vi "Konfig Leak Check.vi"() -> ()   [LabVIEW 2020, in "EPA 1065.lvlib" / "Dichtheitstest 1065-345.lvlib"]
uses:
  Dichtheitstest 1065-345.lvlib
  VFS Button.ctl
  HL Button.ctl
  Versa Button.ctl
  Visualisierungs Elemente/Zahlen-Ausgabefeld.ctl
  Leak Protokoll Einstellungen.ctl
  Seiten/System Einstellungen V2/Analysatoren.ctl
  Aktion Leak Daten.ctl
  Aktion Leak check durchfuehren.ctl
  Aktion Protokolldaten_Leak check.ctl
  Sprachverwaltung/FGV Aktion Tabelle zerlegen.ctl
  Aktion FGV Automatic start.ctl
  Allgemeine VIs/Aktion Wertaenderung Gasliste.ctl
  Allgemeine VIs/Aktion Test Status.ctl
  PNS/Aktionen FGV Grenzwerte.ctl
  Funktionstasten/Zustaende.ctl
  Allgemein/allgemeine Sub-VIs.lvlib
  PNS/PNS.lvlib
  Funktionstasten/Funktionstasten.lvlib
  Sprachverwaltung/Sprachverwaltung.lvlib
  EPA 1065.lvlib
  Linearisierung V2/Protokoll/Protokoll.lvlib
  Seiten/System Einstellungen V2/System Einstellungen V2.lvlib
panel:
  out "Einheit Ergebnis":string caption="Einheit"
  out "Einheit Grenze":string caption="Einheit"
  in  "Einheit":enum16{"mol/s", "mbar"}(ring) caption="Unit:"
  in  "LeakValve":u16(ring) caption="Leak Valve:" items=["inactive", "active"]
  in  "Systemeinstellung":bool caption="Gasliste geändert"
  in  "Save to file":bool caption="Speichern"
  in  "Werte Speichern":bool
  in  "Heizleitung zum VFS":bool caption="Heizleitung\nzum\nVFS"
  in  "HL zu VFS button":T1
  in  "Länge HL zu SP":sgl caption="mm" format="%#.5f"
  in  "Innendurchmesser \nHL zu SP":sgl caption="mm" format="%#.5f"
  in  "Gesamtvolumen VFS":sgl caption="mm³" format="%#.5f"
  in  "Länge HL zu VFS":sgl caption="mm" format="%#.5f"
  in  "Innendurchmesser \nHL zu VFS":sgl caption="mm" format="%#.5f"
  in  "Gesamtvolumen FAS":sgl caption="mm³" format="%#.5f"
  in  "Heizleitung zur Entnahmestelle":bool caption="Heizleitung\nzur\nEntnahmestelle"
  in  "VFS":bool
  in  "HL zu SP button":T1
  in  "VFS button":T2
  out "Anzeige":string
  out "Ergebnis":sgl format="%#.8f"
  out "Grenzwert":sgl format="%#.8f"
  in  "Abbrechen":bool
  in  "Start":bool
  out "Druckanstieg:":T3 caption="mbar"
  out "Druck FT-IR:":T3 caption="atm" format="%.3f"
  out "Status:":string
  in  "Textname:":string
  in  "Pfad:":path=path "D:/IAG_Data"
  in  "PDF speichern":bool caption="Speichern"
  in  "Leak Protokoll":T4={"Bearbeiter:"="", "Pfad:"=path "D:/IAG_Data/Log", "Textname:"="", "Analysator"=""}
  in  "FAS button":T6
  # "Volumen-Einstellungen"
  # "Status"
  # "Druck FT-IR:"
  # "Druckanstieg:"
  # "Innendurchmesser \nHL zu VFS"
  # "Innendurchmesser \nHL zu SP"
  # "Gesamtvolumen Versa"
  # "Gesamtvolumen VFS"
  # "Länge HL zu VFS"
  # "Länge HL zu SP"
  # "Dichtheitstest EPA CRF40 §1065.345"
  # "Protokolleinstellungen"
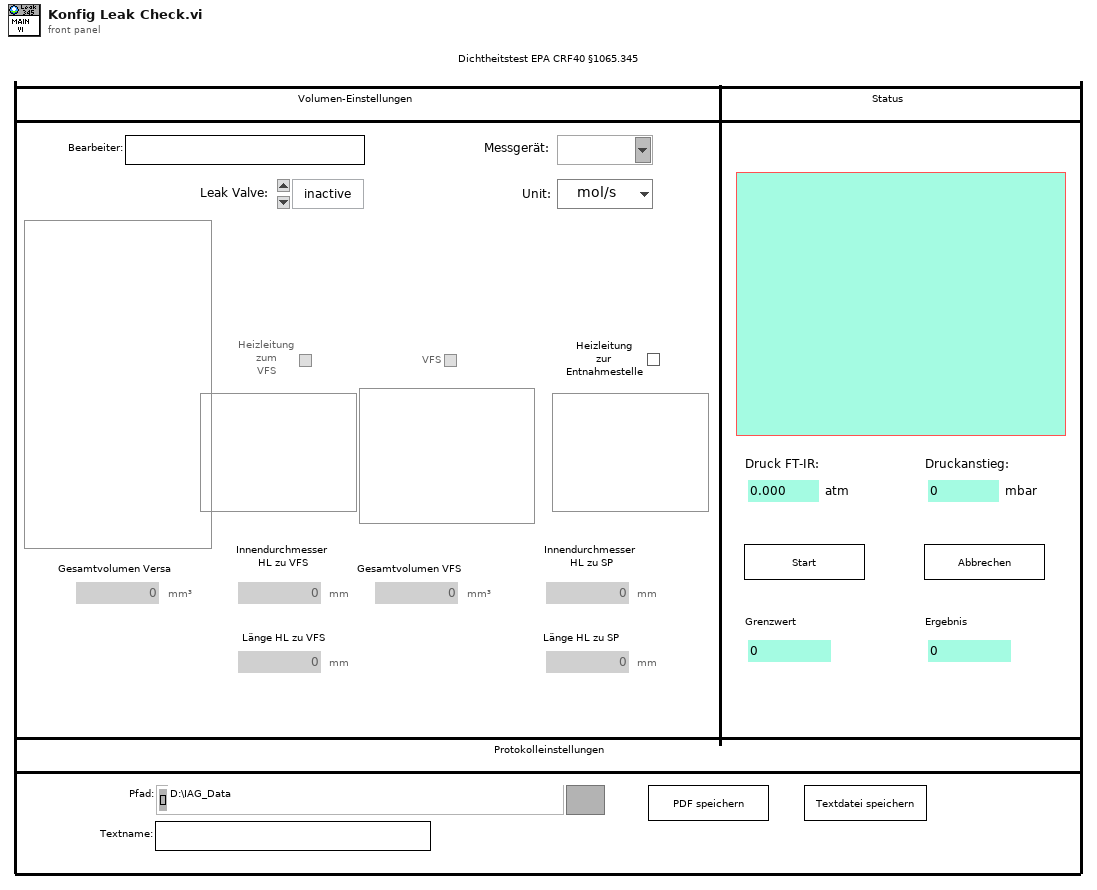
[diagram p1: front panel]
types:
  T1 = typedef "EPA 1065.lvlib/Dichtheitstest 1065-345.lvlib/HL Button.ctl" = bool
  T2 = typedef "EPA 1065.lvlib/Dichtheitstest 1065-345.lvlib/VFS Button.ctl" = bool
  T3 = typedef "Zahlen-Ausgabefeld.ctl" = sgl
  T4 = typedef "EPA 1065.lvlib/Dichtheitstest 1065-345.lvlib/Leak Protokoll Einstellungen.ctl" = cluster{"Bearbeiter:":string, "Pfad:":path, "Textname:":string, "Analysator":T5}
  T5 = typedef "System Einstellungen V2.lvlib/Analysatoren.ctl" = string
  T6 = typedef "EPA 1065.lvlib/Dichtheitstest 1065-345.lvlib/Versa Button.ctl" = bool
  T7 = typedef "Sprachverwaltung.lvlib/FGV Aktion Tabelle zerlegen.ctl" = enum16{"laden", "vereinzeln", "speichern"}
  T8 = typedef "EPA 1065.lvlib/Dichtheitstest 1065-345.lvlib/Aktion Protokolldaten_Leak check.ctl" = enum16{"lesen", "Zeitstempel", "Bearbeiter", "Daten", "Auswertung", "löschen"}
  T9 = typedef "EPA 1065.lvlib/Dichtheitstest 1065-345.lvlib/Aktion Leak Daten.ctl" = enum16{"lesen", "laden", "speichern", "Volumen", "berechnen", "Leak check aktiv", "Leak Zustand", "Pfad", "Pfad speichern"}
  T10 = typedef "EPA 1065.lvlib/Dichtheitstest 1065-345.lvlib/Aktion Leak check durchfuehren.ctl" = enum16{"initialisieren", "Unterdruck erzeugen", "Ventile schließen", "Warten", "Auswertung", "fertig", "PDF erstellen", "abbrechen"}
  T11 = enum8{"Enabled", "Disabled", "Disabled and Grayed Out"}
  T12 = typedef "EPA 1065.lvlib/Dichtheitstest 1065-345.lvlib/Aktion FGV Automatic start.ctl" = enum16{"lesen", "Test starten aktiv", "Test starten inaktiv", "Seite merken", "Seite zurücksetzen", "AK Start inaktiv"}
  T13 = typedef "EPA 1065.lvlib/Dichtheitstest 1065-345.lvlib/Gesamtvolumen.ctl" = cluster{"FAS":sgl, "d von HL zu VFS":sgl, "l von HL zu VFS":sgl, "VFS":sgl, "d von HL zu SP":sgl, "l von HL zu SP":sgl, "Heizleitung zum VFS":bool, "VFS a":bool, "Heizleitung zur Entnahmestelle":bool, "Gesamtes Volumen":sgl, "LeakValve":u16, "Einheit":enum16{"mol/s", "mbar"}}
  T14 = typedef "EPA 1065.lvlib/Aktion Wertaenderung Gasliste.ctl" = enum16{"Init", "lesen", "Gasliste geändert", "ARN inaktiv", "LEAK inaktiv", "Interference 366 inaktiv", "T90 inaktiv", "Interference 375 inaktiv", "Chiller inaktiv", "FID O2 inaktiv", "FID Opti inaktiv", "Drift inaktiv", "Pre Test inaktiv", "LinV2 inaktiv", "HovaCAL Interference inaktiv"}
  T15 = typedef "EPA 1065.lvlib/Aktion Test Status.ctl" = enum16{"init", "lesen", "prüfen", "Interference 366", "Interference 375", "Chiller läuft", "Drift läuft", "Pre Test läuft", "FID Optimization läuft", "FID Interference läuft", "HovaCAL Interference", "LinV2"}
  T16 = enum16{"open", "replace", "create", "open or create", "replace or create", "replace or create with confirmation"}
  T17 = typedef "Funktionstasten.lvlib/Zustaende.ctl" = enum16{"Standby", "Pause", "Eco", "Messen", "Kalibrieren", "Spülen Filter", "Spülen Leitung", "Umgebungsluft", "0-Gas", "Cal-Gas", "CG zu PNS", "-------------", "Init 1", "Init 2", "Init 3", "Init 4", "Messen vorbereiten", "Messen durchführen", "Exit"}
  T18 = typedef "PNS.lvlib/Aktionen FGV Grenzwerte.ctl" = enum16{"lesen", "Grenzw. schreiben", "Anweisungscode", "IP-Adresse", "laden", "speichern", "Anweisungscode vorgeben"}
  T19 = typedef "EPA 1065.lvlib/Dichtheitstest 1065-345.lvlib/Leak Daten.ctl" = cluster{"Gesamtes Volumen":sgl, "p 1":sgl, "p 2":sgl, "T 1":sgl, "T 2":sgl, "t 1":timestamp, "t 2":timestamp, "Ergebnis mol/s":sgl, "Grenze mol/s":sgl, "Leak in %":sgl, "Ergebnis mbar":sgl, "Grenze mbar":sgl}
  T20 = typedef "EPA 1065.lvlib/Aktive Tests Cluster.ctl" = cluster{"ANR läuft":bool, "T90 läuft":bool, "Leak läuft":bool, "Interference 366 läuft":bool, "Interference 375 läuft":bool, "Chiller läuft":bool, "FID Interference läuft":bool, "FID optimization läuft":bool, "Drift läuft":bool, "Pre-test läuft":bool, "HovaCAL Interference läuft":bool, "LinV2 läuft":bool}
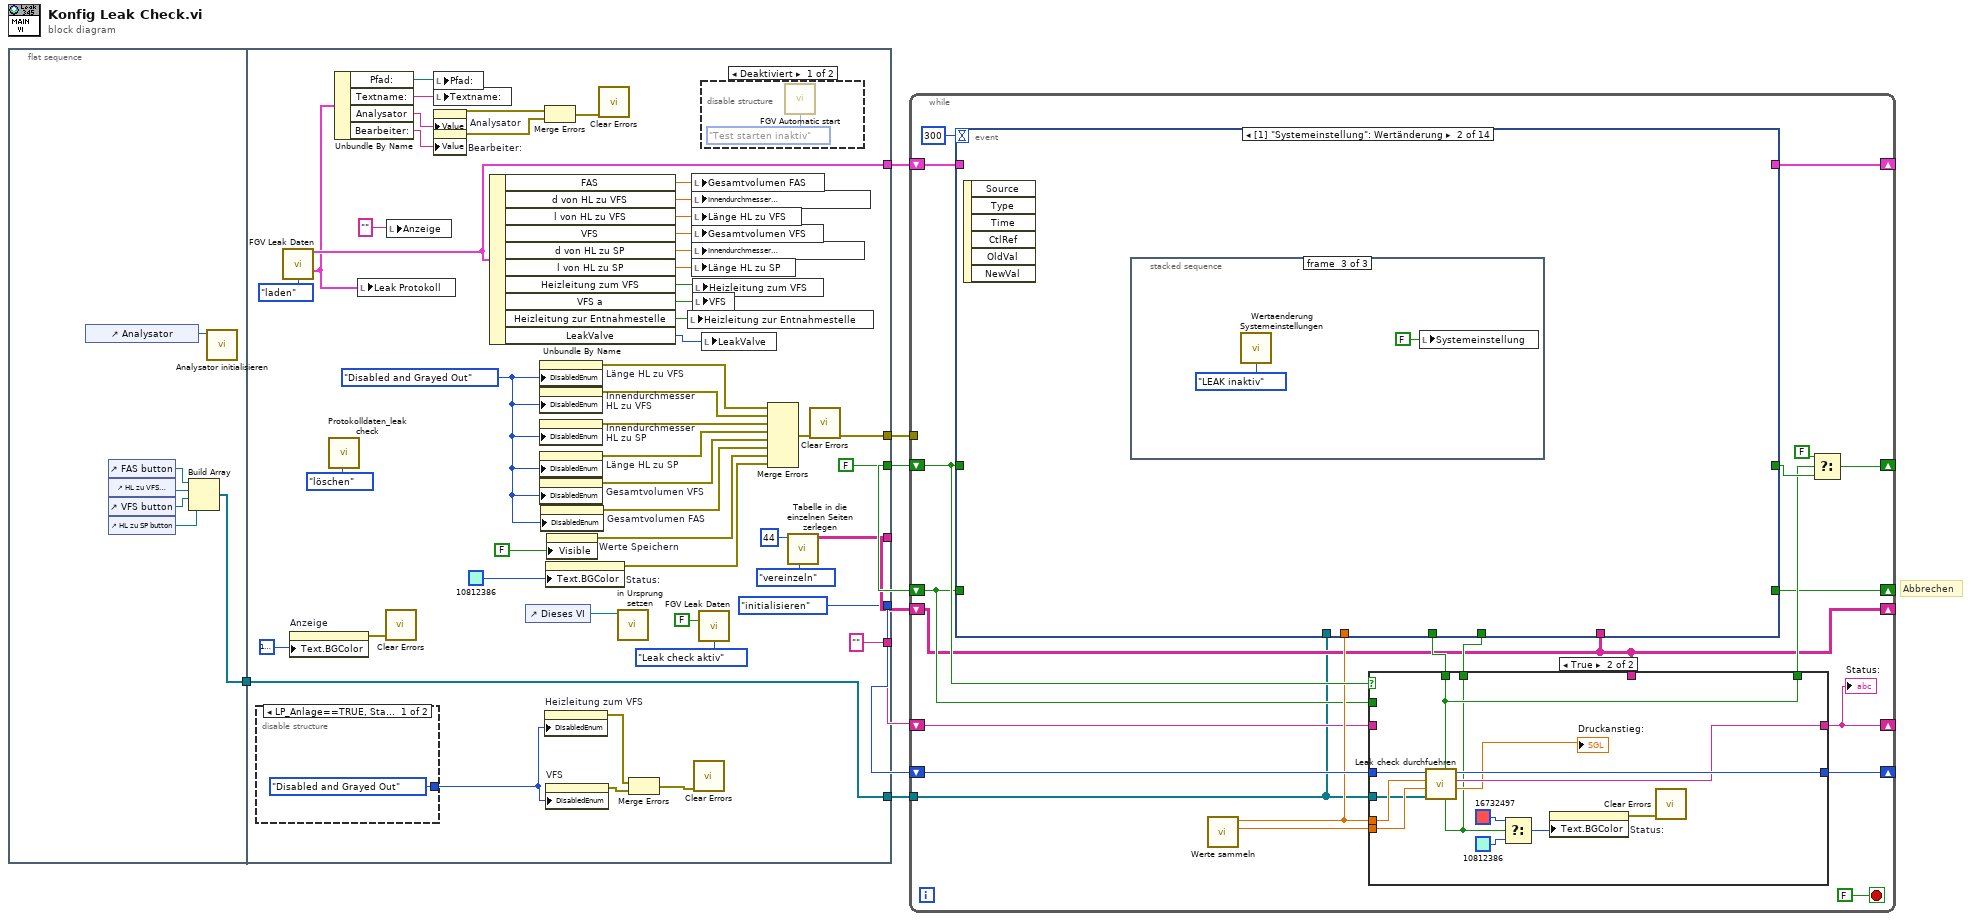
[diagram p0: block diagram]
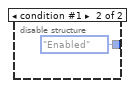
[diagram p2: hidden frame]
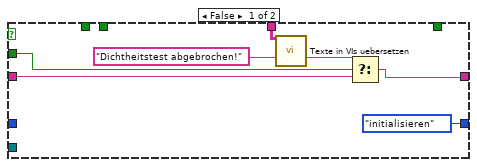
[diagram p4: hidden frame]
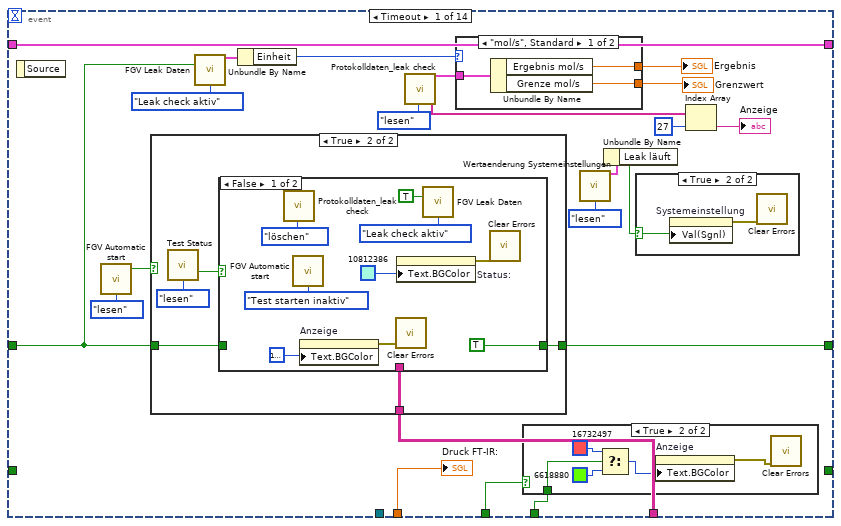
[diagram p5: hidden frame]
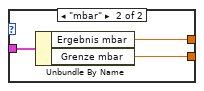
[diagram p6: hidden frame]
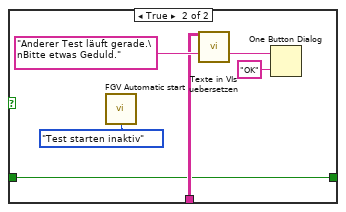
[diagram p9: hidden frame]
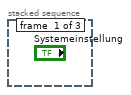
[diagram p11: hidden frame]
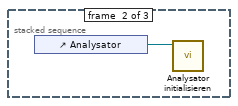
[diagram p12: hidden frame]
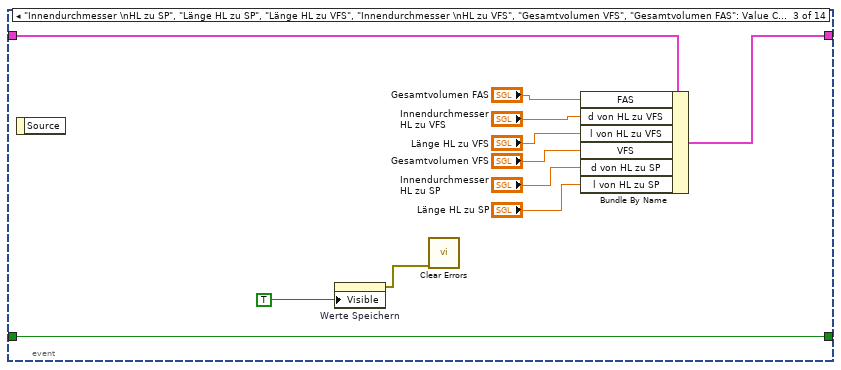
[diagram p13: hidden frame]
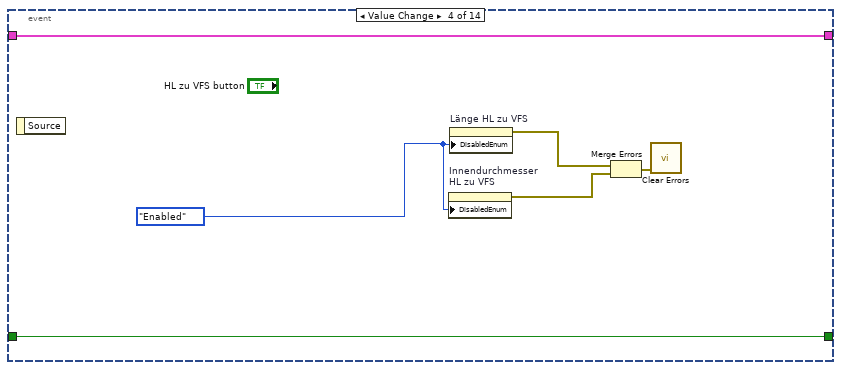
[diagram p14: hidden frame]
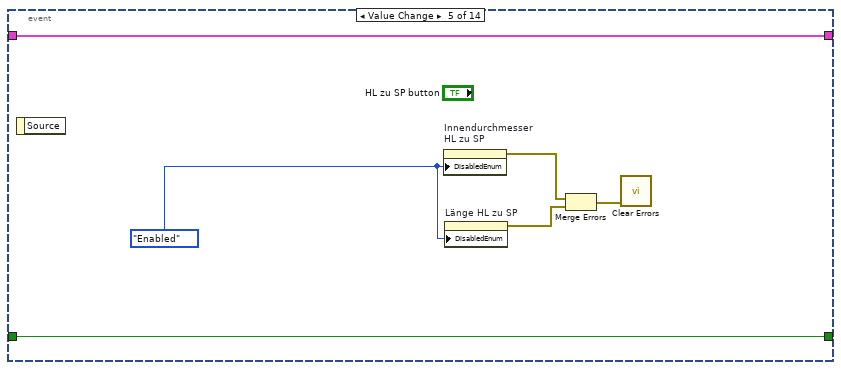
[diagram p15: hidden frame]
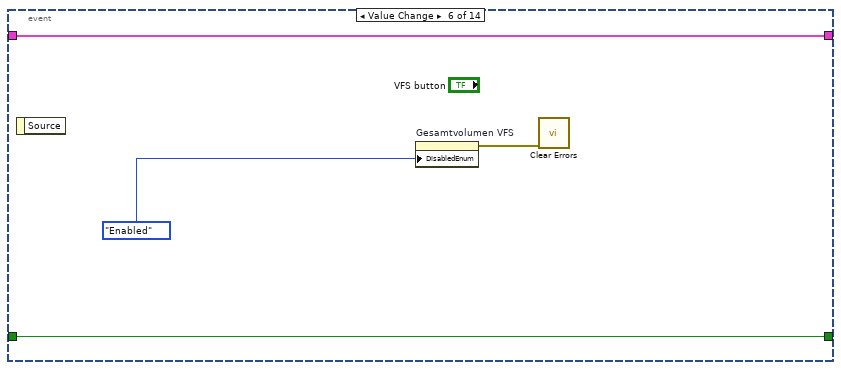
[diagram p16: hidden frame]
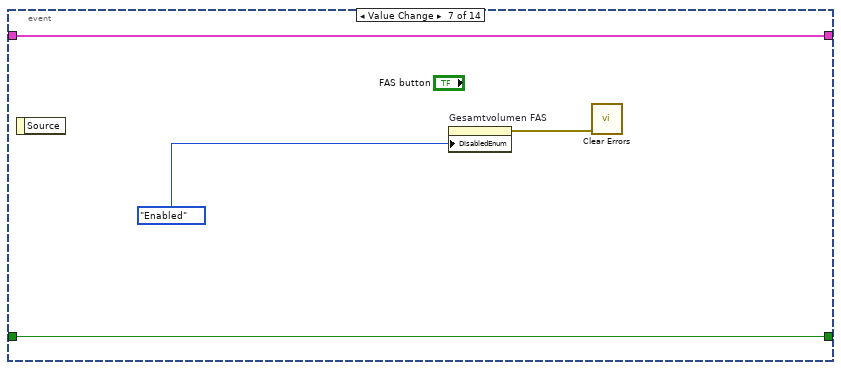
[diagram p17: hidden frame]
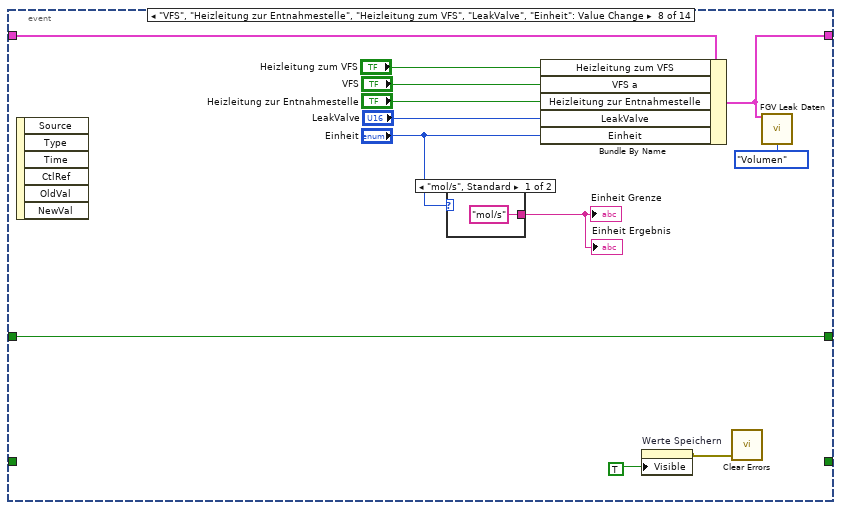
[diagram p18: hidden frame]
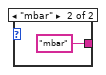
[diagram p19: hidden frame]
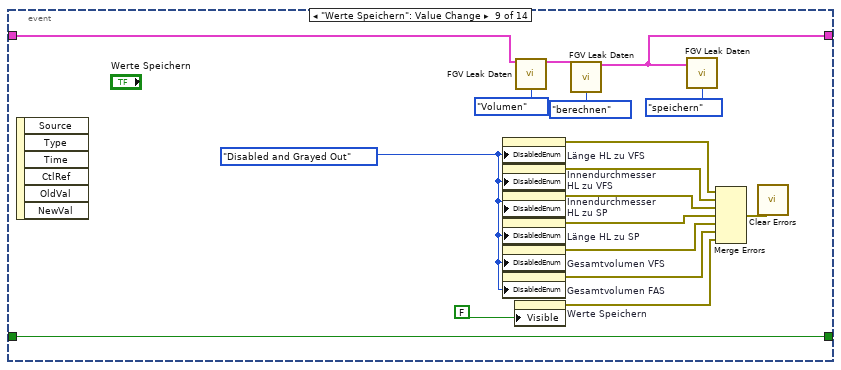
[diagram p20: hidden frame]
diagram:
  # "Abbrechen"
  n1 = flat-sequence {
    tunnel: [w9] -> w2
    tunnel: [w59] -> w8
    tunnel: [w46] -> w7
    tunnel: [FALSE] -> w4
    tunnel: [Aktion_Leak_check_durchfuehren."initialisieren" ("Aktion")] -> w6
    tunnel: ["" ("Status")] -> w5
    tunnel: [w32] -> w3
    tunnel: w2 -> [w15]
    tunnel: [w15] -> w1
    frame #0 {
      n2 = control-ref of="Analysator"() -> (w14:refnum<vi>)
      n3 = control-ref of="FAS button"() -> (w13:refnum<vi>)
      n4 = control-ref of="HL zu VFS button"() -> (w12:refnum<vi>)
      n5 = control-ref of="VFS button"() -> (w11:refnum<vi>)
      n6 = control-ref of="HL zu SP button"() -> (w10:refnum<vi>)
      n7 = Build Array(w13, w12, w11, w10) -> (w9:refnum<vi>[])
      n8 = call "Analysator initialisieren.vi"("Referenz Analysator"=w14) -> ()  [unwired: 9 in, 2 out]
    }
    frame #1 {
      w38 = T11."Disabled and Grayed Out" ("Deaktiviert")
      n9 = disable-structure shown="LP_Anlage==TRUE, Standard" {
        disable-tunnel: [T11."Disabled and Grayed Out" ("Deaktiviert") T11."Enabled" ("Deaktiviert")] -> w20
        frame condition #0 (active) {
        }
        frame condition #1 {
        }
      }
      n10 = call "FGV Leak Daten.vi"("Aktion"=Aktion_Leak_Daten."laden") -> ("Gesamtvolumen"=w46:T13, "Leak Protokoll"=w28:T4)  [unwired: 10 in, 3 out]
      n11 = property on="Anzeige" class="Str"("Text.BGColor"=u32 16777216) -> (error out=w34:errorcluster)  [unwired: 2 in, 1 out]
      n12 = call "Protokolldaten_leak check.vi"("Aktion"=Aktion_Protokolldaten_Leak_check."löschen") -> ()  [unwired: 23 in, 4 out]
      n13 = Unbundle By Name(w28) -> ("Pfad:"=w27:path, "Textname:"=w26:string, "Analysator"=w25:T5, "Bearbeiter:"=w24:string)
      n14 = local write "Leak Protokoll"(w28) -> ()
      n15 = call <vilib>:"Clear Errors.vi"("error in (no error)"=w34) -> ()  [unwired: 5 in, 2 out]
      n16 = local write "Anzeige"("" ("Anzeige")) -> ()
      n17 = local write "Pfad:"(w27) -> ()
      n18 = local write "Textname:"(w26) -> ()
      n19 = property on="Analysator" class="KombiFeld (strikt)"("Value"=w25) -> (error out=w22:errorcluster)  [unwired: 2 in, 1 out]
      n20 = property on="Bearbeiter:" class="Str"("Value"=w24) -> (error out=w21:errorcluster)  [unwired: 2 in, 1 out]
      n21 = Unbundle By Name(w46) -> ("FAS"=w55:sgl, "d von HL zu VFS"=w53:sgl, "l von HL zu VFS"=w52:sgl, "VFS"=w51:sgl, "d von HL zu SP"=w50:sgl, "l von HL zu SP"=w54:sgl, "Heizleitung zum VFS"=w48:bool, "VFS a"=w47:bool, "Heizleitung zur Entnahmestelle"=w49:bool, "LeakValve"=w16:u16)
      n22 = control-ref of="Dieses VI"() -> (w57:refnum<vi>)
      n23 = property on="Länge HL zu VFS" class="DigWert (strikt)"("DisabledEnum"=w38) -> (error out=w64:errorcluster)  [unwired: 2 in, 1 out]
      n24 = property on="Innendurchmesser \nHL zu VFS" class="DigWert (strikt)"("DisabledEnum"=w38) -> (error out=w63:errorcluster)  [unwired: 2 in, 1 out]
      n25 = property on="Innendurchmesser \nHL zu SP" class="DigWert (strikt)"("DisabledEnum"=w38) -> (error out=w62:errorcluster)  [unwired: 2 in, 1 out]
      n26 = property on="Länge HL zu SP" class="DigWert (strikt)"("DisabledEnum"=w38) -> (error out=w61:errorcluster)  [unwired: 2 in, 1 out]
      n27 = property on="Gesamtvolumen VFS" class="DigWert (strikt)"("DisabledEnum"=w38) -> (error out=w60:errorcluster)  [unwired: 2 in, 1 out]
      n28 = property on="Gesamtvolumen FAS" class="DigWert (strikt)"("DisabledEnum"=w38) -> (error out=w58:errorcluster)  [unwired: 2 in, 1 out]
      n29 = Merge Errors(w22, w21) -> (w23:errorcluster)
      n30 = property on="Heizleitung zum VFS" class="Bool. (strikt)"("DisabledEnum"=w20) -> (error out=w18:errorcluster)  [unwired: 2 in, 1 out]
      n31 = property on="Status:" class="Str"("Text.BGColor"=u32 10812386 ("Hintergrund")) -> (error out=w39:errorcluster)  [unwired: 2 in, 1 out]
      n32 = property on="VFS" class="Bool. (strikt)"("DisabledEnum"=w20) -> (error out=w19:errorcluster)  [unwired: 2 in, 1 out]
      n33 = property on="Werte Speichern" class="Bool."("Visible"=FALSE ("Sichtbar")) -> (error out=w30:errorcluster)  [unwired: 2 in, 1 out]
      n34 = call <vilib>:"Clear Errors.vi"("error in (no error)"=w23) -> ()  [unwired: 5 in, 2 out]
      n35 = call "in Ursprung setzen.vi"("VI Referenz"=w57) -> ()  [unwired: 10 in, 1 out]
      n36 = Merge Errors(w18, w19) -> (w17:errorcluster)
      n37 = local write "Heizleitung zur Entnahmestelle"(w49) -> ()
      n38 = local write "Gesamtvolumen FAS"(w55) -> ()
      n39 = local write "Innendurchmesser \nHL zu VFS"(w53) -> ()
      n40 = local write "Länge HL zu VFS"(w52) -> ()
      n41 = local write "Gesamtvolumen VFS"(w51) -> ()
      n42 = local write "Innendurchmesser \nHL zu SP"(w50) -> ()
      n43 = local write "Länge HL zu SP"(w54) -> ()
      n44 = local write "Heizleitung zum VFS"(w48) -> ()
      n45 = local write "VFS"(w47) -> ()
      n46 = call <vilib>:"Clear Errors.vi"("error in (no error)"=w17) -> ()  [unwired: 5 in, 2 out]
      n47 = call "FGV Leak Daten.vi"("Dichtheitstest aktiv"=FALSE, "Aktion"=Aktion_Leak_Daten."Leak check aktiv") -> ()  [unwired: 9 in, 5 out]
      n48 = disable-structure shown="Deaktiviert" {
        frame Disabled {
          n49 = call "FGV Automatic start.vi"("Aktion"=Aktion_FGV_Automatic_start."Test starten inaktiv") -> ()  [unwired: 12 in, 3 out]
        }
        frame Enabled {
        }
      }
      n50 = local write "LeakValve"(w16) -> ()
      n51 = Merge Errors(w64, w63, w62, w61, w60, w58, w30, w39) -> (w65:errorcluster)
      n52 = call "Tabelle in die einzelnen Seiten zerlegen.vi"("Aktion"=FGV_Aktion_Tabelle_zerlegen."vereinzeln", "Index (Seite)"=44) -> ("Sprachliste"=w32:string[][])  [unwired: 7 in, 2 out]
      n53 = call <vilib>:"Clear Errors.vi"("error in (no error)"=w65) -> ("error out"=w59:errorcluster)  [unwired: 5 in, 1 out]
    }
  }
  n54 = while {
    tunnel: w8 -> [_]
    shift-right: [w86] -> _
    shift-left: w7 -> [w87]
    shift-right: [w77] -> _
    shift-left: w4 -> [w85]
    shift-right: [w82] -> _
    shift-left: w6 -> [w83]
    shift-right: [w80] -> _
    shift-left: w5 -> [w79]
    shift-right: [w74] -> _
    shift-left: w4 -> [w73]
    shift-right: [w70] -> _
    shift-left: w3 -> [w70]
    tunnel: w1 -> [w69]
    stop <- FALSE stop-if-true
    n55 = call "Werte sammeln.vi"() -> ("Temperatur"=w84:sgl, "Druck FTIR"=w81:sgl)  [unwired: 10 in]
    n56 = case shown="True" w85 {
      tunnel: w81 -> [_ w109]
      tunnel: w84 -> [_ w108]
      tunnel: w83 -> [_ w107]
      tunnel: [Aktion_Leak_check_durchfuehren."initialisieren" ("Aktion") w106] -> w82
      tunnel: [w94 w105] -> w80
      tunnel: w79 -> [w93 _]
      tunnel: w73 -> [w95 _]
      tunnel: [_ w100] -> w75
      tunnel: [_ w100] -> w72
      tunnel: [_ w98] -> w71
      tunnel: w70 -> [w90 _]
      tunnel: w69 -> [_ w97]
      frame False {
        n57 = call "Texte in VIs uebersetzen.vi"("Sprachliste"=w90, "String zum Übersetzen"="Dichtheitstest abgebrochen!" ("t")) -> ("String zum Übersetzen"=w91:string)  [unwired: 9 in, 4 out]
        n58 = Select(t=w91, s=w95, f=w93) -> (s? t:f=w94:string)
      }
      frame True {
        n59 = call "Leak check durchfuehren.vi"("TablePictures Refnum In"=w97, "Temperatur"=w108, "Druck FT-IR"=w109, "Aktion"=w107) -> ("Druckanstieg"=→"Druckanstieg:":sgl, "Status"=w105:string, "Aktion"=w106:T10, "Fehler"=w98:bool, "Fertig"=w100:bool)  [unwired: 2 in, 1 out]
        n60 = Select(t=u32 16732497 ("Hintergrund"), s=w98, f=u32 10812386 ("Hintergrund")) -> (s? t:f=w102:u32)
        n61 = property on="Status:" class="Str"("Text.BGColor"=w102) -> (error out=w101:errorcluster)  [unwired: 2 in, 1 out]
        n62 = call <vilib>:"Clear Errors.vi"("error in (no error)"=w101) -> ()  [unwired: 5 in, 2 out]
      }
    }
    "Status:" <- w80
    n63 = event shown="[1] \"Systemeinstellung\": Wertänderung" {
      selector: _ -> [_ _ _ _ _ _ _ _ _ _ _ _ _ _]
      dyn-events: _ -> [_ _ _ _ _ _ _ _ _ _ _ _ _ _]
      timeout: 300 -> [_ _ _ _ _ _ _ _ _ _ _ _ _ _]
      tunnel: w87 -> [w129 _ w179 w182 w188 w194 w198 w211 w228 w246 w267 w293 w300 w322]
      tunnel: [w129 _ w178 w182 w188 w194 w198 w205 w218 w246 w267 w293 w300 w322] -> w86
      tunnel: w85 -> [w118 _ w171 w181 w187 w193 w197 w207 w217 w247 w266 w295 _ w320]
      tunnel: [w120 _ w171 w181 w187 w193 w197 w207 w217 w247 w266 w295 w299 w321] -> w78
      tunnel: w81 -> [w131 _ _ _ _ _ _ _ _ _ _ _ _ _]
      tunnel: [_ _ _ _ _ _ _ _ _ w248 w265 w294 _ w319] -> w74
      tunnel: w73 -> [_ _ _ _ _ _ _ _ _ w248 w265 w294 _ _]
      tunnel: w72 -> [w124 _ _ _ _ _ _ _ _ _ _ _ _ _]
      tunnel: w71 -> [w123 _ _ _ _ _ _ _ _ _ _ _ _ _]
      tunnel: w70 -> [w119 _ _ _ _ _ _ _ _ _ _ _ w296 _]
      tunnel: w69 -> [_ _ _ _ _ _ _ _ _ w231 _ _ _ _]
      event Timeout {
        n64 = event-data() -> ()  [unwired: 1 in, 1 out]
        n65 = call "FGV Automatic start.vi"("Aktion"=Aktion_FGV_Automatic_start."lesen") -> ("Starten"=w122:bool)  [unwired: 12 in, 2 out]
        n66 = case shown="True" w122 {
          tunnel: [w140 w143] -> w120
          tunnel: w119 -> [_ w142]
          tunnel: w118 -> [w140 w141]
          frame False {
          }
          frame True {
            n67 = call "Test Status.vi"("Aktion"=Aktion_Test_Status."lesen") -> ("Tests sperren"=w145:bool)  [unwired: 11 in, 3 out]
            n68 = case shown="False" w145 {
              tunnel: [TRUE w156] -> w143
              tunnel: w142 -> [_ w157]
              tunnel: w141 -> [_ w156]
              frame False {
                n69 = call "Protokolldaten_leak check.vi"("Aktion"=Aktion_Protokolldaten_Leak_check."löschen") -> ()  [unwired: 23 in, 4 out]
                n70 = call "FGV Automatic start.vi"("Aktion"=Aktion_FGV_Automatic_start."Test starten inaktiv") -> ()  [unwired: 12 in, 3 out]
                n71 = property on="Anzeige" class="Str"("Text.BGColor"=u32 16777216) -> (error out=w148:errorcluster)  [unwired: 2 in, 1 out]
                n72 = call <vilib>:"Clear Errors.vi"("error in (no error)"=w148) -> ()  [unwired: 5 in, 2 out]
                n73 = property on="Status:" class="Str"("Text.BGColor"=u32 10812386 ("Hintergrund")) -> (error out=w152:errorcluster)  [unwired: 2 in, 1 out]
                n74 = call "FGV Leak Daten.vi"("Dichtheitstest aktiv"=TRUE, "Aktion"=Aktion_Leak_Daten."Leak check aktiv") -> ()  [unwired: 9 in, 5 out]
                n75 = call <vilib>:"Clear Errors.vi"("error in (no error)"=w152) -> ()  [unwired: 5 in, 2 out]
              }
              frame True {
                n76 = call "FGV Automatic start.vi"("Aktion"=Aktion_FGV_Automatic_start."Test starten inaktiv") -> ()  [unwired: 12 in, 3 out]
                n77 = call "Texte in VIs uebersetzen.vi"("Sprachliste"=w157, "String zum Übersetzen"="Anderer Test läuft gerade.\nBitte etwas Geduld." ("Nachricht")) -> ("String zum Übersetzen"=w158:string)  [unwired: 9 in, 4 out]
                n78 = One Button Dialog(message=w158, button name ("OK")="OK" ("Schaltflächentext (\"OK\")")) -> ()  [unwired: 1 out]
              }
            }
          }
        }
        n79 = call "FGV Leak Daten.vi"("Dichtheitstest aktiv"=w118, "Aktion"=Aktion_Leak_Daten."Leak check aktiv") -> ("Gesamtvolumen"=w113:T13)  [unwired: 9 in, 4 out]
        n80 = Unbundle By Name(w113) -> ("Einheit"=w112:enum16{"mol/s", "mbar"})
        n81 = call "Protokolldaten_leak check.vi"("Aktion"=Aktion_Protokolldaten_Leak_check."lesen") -> ("Auswertung"=w127:string[], "Daten"=w114:T19)  [unwired: 23 in, 2 out]
        n82 = case shown="\"mol/s\", Standard" w112 {
          tunnel: w114 -> [w134 w137]
          tunnel: [w133 w136] -> w111
          tunnel: [w132 w135] -> w110
          frame "mol/s", Default {
            n83 = Unbundle By Name(w134) -> ("Ergebnis mol/s"=w133:sgl, "Grenze mol/s"=w132:sgl)
          }
          frame "mbar" {
            n84 = Unbundle By Name(w137) -> ("Ergebnis mbar"=w136:sgl, "Grenze mbar"=w135:sgl)
          }
        }
        "Grenzwert" <- w110
        "Ergebnis" <- w111
        n85 = case shown="True" w124 {
          tunnel: w123 -> [_ w163]
          frame False {
          }
          frame True {
            n86 = Select(t=u32 16732497 ("Hintergrund"), s=w163, f=u32 6618880 ("Hintergrund")) -> (s? t:f=w162:u32)
            n87 = property on="Anzeige" class="Str"("Text.BGColor"=w162) -> (error out=w161:errorcluster)  [unwired: 2 in, 1 out]
            n88 = call <vilib>:"Clear Errors.vi"("error in (no error)"=w161) -> ()  [unwired: 5 in, 2 out]
          }
        }
        n89 = call "Wertaenderung Systemeinstellungen.vi"("Aktion"=Aktion_Wertaenderung_Gasliste."lesen") -> ("Tests"=w116:T20)  [unwired: 13 in, 1 out]
        n90 = Unbundle By Name(w116) -> ("Leak läuft"=w115:bool)
        n91 = case shown="True" w115 {
          selector: w115 -> [_ w139]
          frame False {
          }
          frame True {
            n92 = property on="Systemeinstellung" class="Bool. (strikt)"("Val(Sgnl)"=w139) -> (error out=w138:errorcluster)  [unwired: 2 in, 1 out]
            n93 = call <vilib>:"Clear Errors.vi"("error in (no error)"=w138) -> ()  [unwired: 5 in, 2 out]
          }
        }
        n94 = Index Array(array=w127, index=27 ("Index")) -> (element=→"Anzeige":string)
        "Druck FT-IR:" <- w131
      }
      event "Systemeinstellung": Value Change {
        n95 = event-data() -> ()  [unwired: 1 in, 6 out]
        n96 = stacked-sequence {
          frame #0 {
          }
          frame #1 {
            n97 = control-ref of="Analysator"() -> (w166:refnum<vi>)
            n98 = call "Analysator initialisieren.vi"("Referenz Analysator"=w166) -> ()  [unwired: 9 in, 2 out]
          }
          frame #2 {
            n99 = call "Wertaenderung Systemeinstellungen.vi"("Aktion"=Aktion_Wertaenderung_Gasliste."LEAK inaktiv") -> ()  [unwired: 13 in, 2 out]
            n100 = local write "Systemeinstellung"(FALSE ("Systemeinstellung")) -> ()
          }
        }
      }
      event "Innendurchmesser \nHL zu SP", "Länge HL zu SP", "Länge HL zu VFS", "Innendurchmesser \nHL zu VFS", "Gesamtvolumen VFS", "Gesamtvolumen FAS": Value Change {
        n101 = event-data() -> ()  [unwired: 1 in, 1 out]
        n102 = property on="Werte Speichern" class="Bool."("Visible"=TRUE ("Sichtbar")) -> (error out=w169:errorcluster)  [unwired: 2 in, 1 out]
        n103 = call <vilib>:"Clear Errors.vi"("error in (no error)"=w169) -> ()  [unwired: 5 in, 2 out]
        n104 = Bundle By Name(cluster=w179, "FAS"="Gesamtvolumen FAS", "d von HL zu VFS"="Innendurchmesser \nHL zu VFS", "l von HL zu VFS"="Länge HL zu VFS", "VFS"="Gesamtvolumen VFS", "d von HL zu SP"="Innendurchmesser \nHL zu SP", "l von HL zu SP"="Länge HL zu SP") -> (w178:T13)
      }
      event Value Change {
        w180 = T11."Enabled" ("Deaktiviert")
        n105 = event-data() -> ()  [unwired: 1 in, 1 out]
        n106 = property on="Innendurchmesser \nHL zu VFS" class="DigWert (strikt)"("DisabledEnum"=w180) -> (error out=w184:errorcluster)  [unwired: 2 in, 1 out]
        n107 = property on="Länge HL zu VFS" class="DigWert (strikt)"("DisabledEnum"=w180) -> (error out=w185:errorcluster)  [unwired: 2 in, 1 out]
        n108 = Merge Errors(w185, w184) -> (w183:errorcluster)
        n109 = call <vilib>:"Clear Errors.vi"("error in (no error)"=w183) -> ()  [unwired: 5 in, 2 out]
      }
      event Value Change {
        w186 = T11."Enabled" ("Deaktiviert")
        n110 = event-data() -> ()  [unwired: 1 in, 1 out]
        n111 = property on="Innendurchmesser \nHL zu SP" class="DigWert (strikt)"("DisabledEnum"=w186) -> (error out=w191:errorcluster)  [unwired: 2 in, 1 out]
        n112 = property on="Länge HL zu SP" class="DigWert (strikt)"("DisabledEnum"=w186) -> (error out=w190:errorcluster)  [unwired: 2 in, 1 out]
        n113 = Merge Errors(w191, w190) -> (w189:errorcluster)
        n114 = call <vilib>:"Clear Errors.vi"("error in (no error)"=w189) -> ()  [unwired: 5 in, 2 out]
      }
      event Value Change {
        n115 = event-data() -> ()  [unwired: 1 in, 1 out]
        n116 = property on="Gesamtvolumen VFS" class="DigWert (strikt)"("DisabledEnum"=T11."Enabled" ("Deaktiviert")) -> (error out=w195:errorcluster)  [unwired: 2 in, 1 out]
        n117 = call <vilib>:"Clear Errors.vi"("error in (no error)"=w195) -> ()  [unwired: 5 in, 2 out]
      }
      event Value Change {
        n118 = event-data() -> ()  [unwired: 1 in, 1 out]
        n119 = property on="Gesamtvolumen FAS" class="DigWert (strikt)"("DisabledEnum"=T11."Enabled" ("Deaktiviert")) -> (error out=w199:errorcluster)  [unwired: 2 in, 1 out]
        n120 = call <vilib>:"Clear Errors.vi"("error in (no error)"=w199) -> ()  [unwired: 5 in, 2 out]
      }
      event "VFS", "Heizleitung zur Entnahmestelle", "Heizleitung zum VFS", "LeakValve", "Einheit": Value Change {
        n121 = event-data() -> ()  [unwired: 1 in, 6 out]
        n122 = case shown="\"mol/s\", Standard" "Einheit" {
          tunnel: ["mol/s" "mbar"] -> w200
          frame "mol/s", Default {
          }
          frame "mbar" {
          }
        }
        "Einheit Grenze" <- w200
        "Einheit Ergebnis" <- w200
        n123 = Bundle By Name(cluster=w211, "Heizleitung zum VFS"="Heizleitung zum VFS", "VFS a"="VFS", "Heizleitung zur Entnahmestelle"="Heizleitung zur Entnahmestelle", "LeakValve"="LeakValve", "Einheit"="Einheit") -> (w205:T13)
        n124 = property on="Werte Speichern" class="Bool."("Visible"=TRUE ("Sichtbar")) -> (error out=w203:errorcluster)  [unwired: 2 in, 1 out]
        n125 = call <vilib>:"Clear Errors.vi"("error in (no error)"=w203) -> ()  [unwired: 5 in, 2 out]
        n126 = call "FGV Leak Daten.vi"("Gesamtvolumen"=w205, "Aktion"=Aktion_Leak_Daten."Volumen") -> ()  [unwired: 9 in, 5 out]
      }
      event "Werte Speichern": Value Change {
        w216 = T11."Disabled and Grayed Out" ("Deaktiviert")
        n127 = event-data() -> ()  [unwired: 1 in, 6 out]
        n128 = property on="Länge HL zu VFS" class="DigWert (strikt)"("DisabledEnum"=w216) -> (error out=w222:errorcluster)  [unwired: 2 in, 1 out]
        n129 = property on="Innendurchmesser \nHL zu VFS" class="DigWert (strikt)"("DisabledEnum"=w216) -> (error out=w223:errorcluster)  [unwired: 2 in, 1 out]
        n130 = property on="Innendurchmesser \nHL zu SP" class="DigWert (strikt)"("DisabledEnum"=w216) -> (error out=w224:errorcluster)  [unwired: 2 in, 1 out]
        n131 = property on="Länge HL zu SP" class="DigWert (strikt)"("DisabledEnum"=w216) -> (error out=w225:errorcluster)  [unwired: 2 in, 1 out]
        n132 = property on="Gesamtvolumen VFS" class="DigWert (strikt)"("DisabledEnum"=w216) -> (error out=w226:errorcluster)  [unwired: 2 in, 1 out]
        n133 = property on="Gesamtvolumen FAS" class="DigWert (strikt)"("DisabledEnum"=w216) -> (error out=w227:errorcluster)  [unwired: 2 in, 1 out]
        n134 = property on="Werte Speichern" class="Bool."("Visible"=FALSE ("Sichtbar")) -> (error out=w214:errorcluster)  [unwired: 2 in, 1 out]
        n135 = call "FGV Leak Daten.vi"("Gesamtvolumen"=w228, "Aktion"=Aktion_Leak_Daten."Volumen") -> ("Gesamtvolumen"=w219:T13)  [unwired: 9 in, 4 out]
        n136 = call "FGV Leak Daten.vi"("Gesamtvolumen"=w219, "Aktion"=Aktion_Leak_Daten."berechnen") -> ("Gesamtvolumen"=w218:T13)  [unwired: 9 in, 4 out]
        n137 = call "FGV Leak Daten.vi"("Gesamtvolumen"=w218, "Aktion"=Aktion_Leak_Daten."speichern") -> ()  [unwired: 9 in, 5 out]
        n138 = Merge Errors(w222, w223, w224, w225, w226, w227, w214) -> (w221:errorcluster)
        n139 = call <vilib>:"Clear Errors.vi"("error in (no error)"=w221) -> ()  [unwired: 5 in, 2 out]
      }
      event "PDF speichern": Value Change {
        n140 = event-data() -> ()  [unwired: 1 in, 1 out]
        n141 = call "FGV Leak Daten.vi"("Aktion"=Aktion_Leak_Daten."lesen") -> ("Leak Protokoll"=w241:T4)  [unwired: 10 in, 4 out]
        n142 = Unbundle By Name(w241) -> ("Pfad:"=w240:path, "Textname:"=w239:string)
        n143 = Concatenate Strings(w239, ".pdf" ("String")) -> (w244:string)
        n144 = Build Path(base path=w240, name or relative path=w244) -> (appended path=w232:path)
        n145 = disable-structure shown="BullZip==TRUE" {
          disable-tunnel: w232 -> [w258 _]
          disable-tunnel: [w257 _] -> w243
          frame condition #0 {
            n146 = call "Save to PDF File using BullZip 2009.vi"("Save PDF File Path"=w258) -> ("error out"=w257:errorcluster)  [unwired: 10 in]
          }
          frame condition #1 (active) {
          }
        }
        n147 = disable-structure shown="Aktiviert" {
          disable-tunnel: w243 -> [w250 w254]
          disable-tunnel: [w249 w253] -> w233
          disable-tunnel: w232 -> [_ w252]
          disable-tunnel: w231 -> [_ w251]
          frame Disabled {
            n148 = call "PDF Protokoll EPA1065_LeakCheck.vi"("error in (no error)"=w250) -> ("error out"=w249:errorcluster)  [unwired: 10 in]
          }
          frame Enabled {
            # "#PDF_Interface"
            n149 = call "PDF_Interface_PDF Protokoll EPA1065_LeakCheck.vi"("error in (no error)"=w254, "TablePictures Refnum In"=w251, "Save PDF File Path"=w252) -> ("error out"=w253:errorcluster)  [unwired: 8 in]
          }
        }
        n150 = case shown="Kein Fehler" w233 {
          tunnel: ["Daten gespeichert!" ("String") "Fehler beim schreiben der Daten" ("String")] -> w236
          frame No Error {
          }
          frame Error {
          }
        }
        n151 = call "Tabelle in die einzelnen Seiten zerlegen.vi"("Aktion"=FGV_Aktion_Tabelle_zerlegen."vereinzeln", "Index (Seite)"=38) -> ("Sprachliste"=w237:string[][])  [unwired: 7 in, 2 out]
        n152 = call "Texte in VIs uebersetzen.vi"("Sprachliste"=w237, "String zum Übersetzen"=w236) -> ("String zum Übersetzen"=w235:string)  [unwired: 9 in, 4 out]
        n153 = One Button Dialog(message=w235) -> ()  [unwired: 1 in, 1 out]
      }
      event "Save to file": Value Change {
        n154 = event-data() -> ()  [unwired: 1 in, 6 out]
        n155 = call "FGV Leak Daten.vi"("Aktion"=Aktion_Leak_Daten."lesen") -> ("Leak Protokoll"=w270:T4)  [unwired: 10 in, 4 out]
        n156 = Unbundle By Name(w270) -> ("Pfad:"=w269:path, "Textname:"=w268:string)
        n157 = Concatenate Strings(w268, ".txt" ("String")) -> (w278:string)
        n158 = call "Protokolldaten_leak check.vi"("Aktion"=Aktion_Protokolldaten_Leak_check."lesen") -> ("Auswertung"=w272:string[])  [unwired: 23 in, 3 out]
        n159 = Build Path(base path=w269, name or relative path=w278) -> (appended path=w279:path)
        n160 = Open/Create/Replace File(file path (use dialog)=w279, operation (0:open)=T16."replace or create with confirmation" ("Operation (0:Öffnen)")) -> (refnum out=w275:refnum<file>, error out=w276:errorcluster)  [unwired: 4 in, 1 out]
        n161 = Write to Text File(file (use dialog)=w275, text=w272, error in=w276) -> (refnum out=w281:refnum<file>, error out=w259:errorcluster)  [unwired: 1 in, 1 out]
        n162 = case shown="Fehler" w259 {
          tunnel: ["Daten gespeichert!" ("String") "Fehler beim schreiben der Daten" ("String")] -> w262
          frame No Error {
          }
          frame Error {
          }
        }
        n163 = Close File(refnum=w281, error in=w259) -> (error out=w280:errorcluster)  [unwired: 1 out]
        n164 = call <vilib>:"Clear Errors.vi"("error in (no error)"=w280) -> ()  [unwired: 5 in, 2 out]
        n165 = call "Tabelle in die einzelnen Seiten zerlegen.vi"("Aktion"=FGV_Aktion_Tabelle_zerlegen."vereinzeln", "Index (Seite)"=38) -> ("Sprachliste"=w263:string[][])  [unwired: 7 in, 2 out]
        n166 = call "Texte in VIs uebersetzen.vi"("Sprachliste"=w263, "String zum Übersetzen"=w262) -> ("String zum Übersetzen"=w261:string)  [unwired: 9 in, 4 out]
        n167 = One Button Dialog(message=w261) -> ()  [unwired: 1 in, 1 out]
      }
      event "Pfad:", "Textname:": Value Change {
        n168 = event-data() -> ()  [unwired: 1 in, 1 out]
        n169 = Unbundle By Name("Leak Protokoll") -> ("Analysator"=w285:T5, "Bearbeiter:"=w284:string)
        n170 = Bundle By Name(cluster="Leak Protokoll", "Pfad:"="Pfad:", "Textname:"="Textname:", "Analysator"=w285, "Bearbeiter:"=w284) -> (w289:T4)
        n171 = call "FGV Leak Daten.vi"("Leak Protokoll"=w289, "Aktion"=Aktion_Leak_Daten."Pfad") -> ("error out"=w290:errorcluster)  [unwired: 9 in, 4 out]
        n172 = call "FGV Leak Daten.vi"("error in (no error)"=w290, "Aktion"=Aktion_Leak_Daten."Pfad speichern") -> ()  [unwired: 9 in, 5 out]
      }
      event "Start": Value Change {
        n173 = event-data() -> ()  [unwired: 1 in, 1 out]
        n174 = call "Test Status.vi"("Aktion"=Aktion_Test_Status."lesen") -> ("Tests sperren"=w297:bool)  [unwired: 11 in, 3 out]
        n175 = case shown="False" w297 {
          tunnel: [TRUE FALSE] -> w299
          tunnel: w296 -> [_ w309]
          frame False {
            n176 = property on="Anzeige" class="Str"("Text.BGColor"=u32 16777216) -> (error out=w302:errorcluster)  [unwired: 2 in, 1 out]
            n177 = call "Protokolldaten_leak check.vi"("Aktion"=Aktion_Protokolldaten_Leak_check."löschen") -> ()  [unwired: 23 in, 4 out]
            n178 = property on="Status:" class="Str"("Text.BGColor"=u32 10812386 ("Hintergrund")) -> (error out=w306:errorcluster)  [unwired: 2 in, 1 out]
            n179 = call <vilib>:"Clear Errors.vi"("error in (no error)"=w302) -> ()  [unwired: 5 in, 2 out]
            n180 = call "FGV Leak Daten.vi"("Dichtheitstest aktiv"=TRUE, "Aktion"=Aktion_Leak_Daten."Leak check aktiv") -> ()  [unwired: 9 in, 5 out]
            n181 = call <vilib>:"Clear Errors.vi"("error in (no error)"=w306) -> ()  [unwired: 5 in, 2 out]
          }
          frame True {
            n182 = call "Texte in VIs uebersetzen.vi"("Sprachliste"=w309, "String zum Übersetzen"="Anderer Test läuft gerade.\nBitte etwas Geduld." ("Nachricht")) -> ("String zum Übersetzen"=w310:string)  [unwired: 9 in, 4 out]
            n183 = One Button Dialog(message=w310, button name ("OK")="OK" ("Schaltflächentext (\"OK\")")) -> ()  [unwired: 1 out]
          }
        }
      }
      event "Abbrechen": Value Change {
        n184 = event-data() -> ()  [unwired: 1 in, 1 out]
        n185 = call "Test Status.vi"("Aktion"=Aktion_Test_Status."lesen") -> ("Aktive Tests"=w317:T20, "Tests sperren"=w315:bool)  [unwired: 11 in, 2 out]
        n186 = Unbundle By Name(w317) -> ("Leak läuft"=w316:bool)
        n187 = And(x=w316, y=w315) -> (x .and. y?=w314:bool)
        n188 = case shown="True" w314 {
          tunnel: [w324 FALSE] -> w321
          tunnel: w320 -> [w324 w325]
          tunnel: [FALSE w325] -> w319
          frame False {
          }
          frame True {
            # "abbrechen damit es wieder freigegeben wird"
            # "Um das Gebläse abzuschalten initialisieren"
            n189 = call "Protokolldaten_leak check.vi"("Aktion"=Aktion_Protokolldaten_Leak_check."löschen") -> ()  [unwired: 23 in, 4 out]
            n190 = call "FGV Leak Daten.vi"("Dichtheitstest aktiv"=FALSE, "Aktion"=Aktion_Leak_Daten."Leak check aktiv") -> ()  [unwired: 9 in, 5 out]
            n191 = call "Leak check durchfuehren.vi"("Aktion"=Aktion_Leak_check_durchfuehren."abbrechen") -> ()  [unwired: 5 in, 6 out]
            n192 = call "FGV Grenzwerte PNS.vi"("Zustand"=Zustaende."Standby", "Aktionen FGV Grenzwerte"=Aktionen_FGV_Grenzwerte."Anweisungscode") -> ()  [unwired: 11 in, 3 out]
          }
        }
      }
    }
    n193 = Select(t=FALSE, s=w75, f=w78) -> (s? t:f=w77:bool)
  }
